vi "Write Vertical Scroll.vi"(8 "error in (no error)":errorcluster, 10 "Horizontal Scroll":T1 caption="Vertical Scroll", 11 "Pane in":refnum<class "Pane.lvclass">) -> (0 "error out":errorcluster, 3 "Pane out":refnum<class "Pane.lvclass">)   [LabVIEW 2017, in "Pane.lvclass"]
uses:
  Pane.lvclass
  Typedefs/Scrollbar Visibility--Enum.ctl
  Pane.lvclass/Pane.ctl
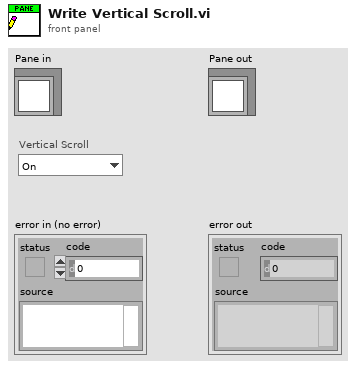
[diagram p1: front panel]
types:
  T1 = typedef "Scrollbar Visibility--Enum.ctl" = enum16{"On", "Off", "Off (Runtime)"}
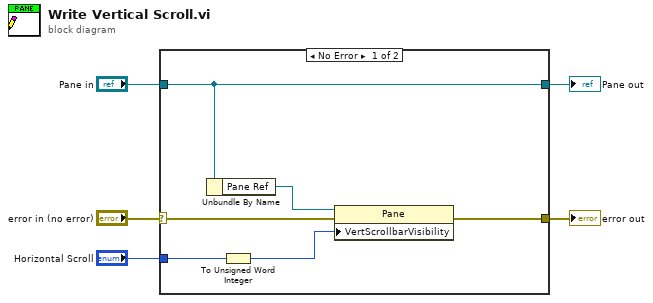
[diagram p0: block diagram]
diagram:
  n1 = case shown="No Error" "error in (no error)" {
    selector: "error in (no error)" -> [w11 w12]
    tunnel: [w10 w12] -> w4
    tunnel: [w8 w13] -> w2
    tunnel: "Pane in" -> [w8 w13]
    tunnel: "Horizontal Scroll" -> [w9 _]
    frame No Error {
      n2 = Unbundle By Name(w8) -> ("Pane Ref"=w7:refnum<vi>)
      n3 = To Unsigned Word Integer(number=w9) -> (unsigned 16bit integer=w6:u16)
      n4 = property class="Pane"(reference=w7, error in=w11, "VertScrollbarVisibility"=w6) -> (error out=w10:errorcluster)  [unwired: 1 out]
    }
    frame Error {
    }
  }
  "error out" <- w4
  "Pane out" <- w2
